vi "CLD 1 Elapsed Time Express Front Panel.vi"() -> ()   [LabVIEW 2017]
doc: "LabVIEW CLD 1 Exercise"
panel:
  out "Elapsed Time (s)":dbl format="%.3g"
  out "error out":errorcluster
  in  "error in":errorcluster
  out "Time has Elapsed":bool
  in  "Auto Reset":bool=TRUE
  in  "Reset Button":bool
  in  "Stop VI":bool
  in  "Time Target (s)":dbl
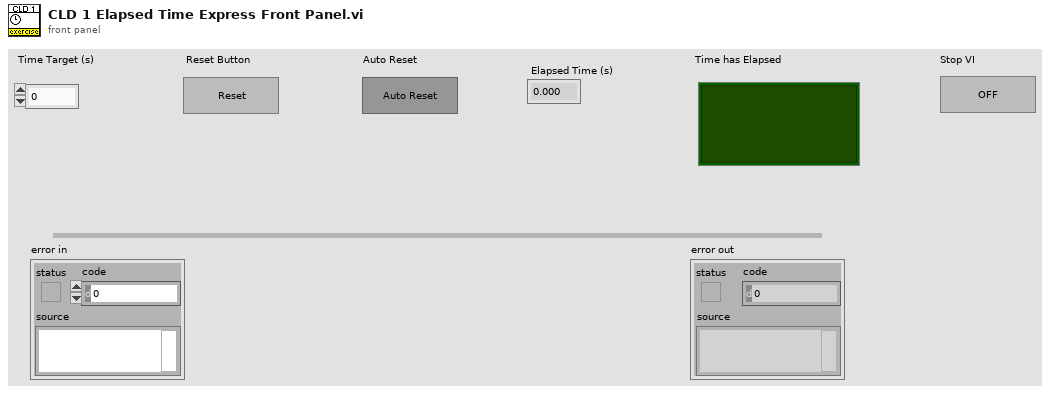
[diagram p1: front panel]
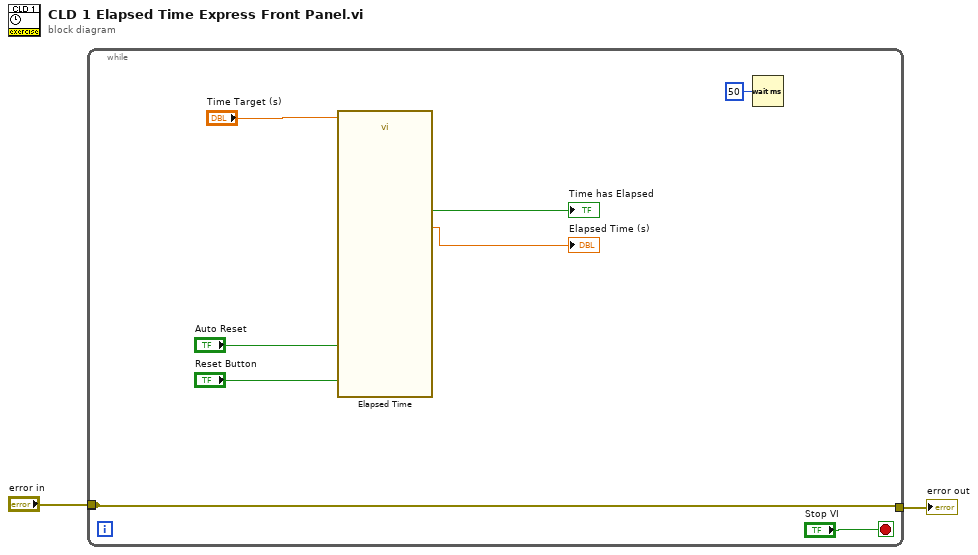
[diagram p0: block diagram]
diagram:
  n1 = while {
    tunnel: [w9] -> _
    tunnel: "error in" -> [w9]
    tunnel: [w9] -> w1
    stop <- "Stop VI" stop-if-true
    n2 = call "Elapsed Time"("Time Target (s)"="Time Target (s)", "Reset"="Reset Button", "Auto Reset"="Auto Reset") -> ("Elapsed Time (s)"=→"Elapsed Time (s)":dbl, "Time has Elapsed"=→"Time has Elapsed":bool)  [unwired: 9 in, 6 out]
    n3 = Wait (ms)(milliseconds to wait=u32 50) -> ()  [unwired: 1 out]
  }
  "error out" <- w1
